vi "characterisation.vi"   [LabVIEW 2019]
uses:
  Shared VIs/ModelSpecific/ETHMikeModel.ctl
  Shared VIs/ModelSpecific/ReadOnlyGlobalActions.ctl
types:
  T1 = typedef "ReadOnlyGlobalActions.ctl" = enum16{"Initialize", "Read", "Write"}
  T2 = typedef "ETHMikeModel.ctl" = enum16{"ETH Mike #1", "ETH Mike #2", "ETH Mike #3", "ETH Mike #4", "ETH MIKE #5"}
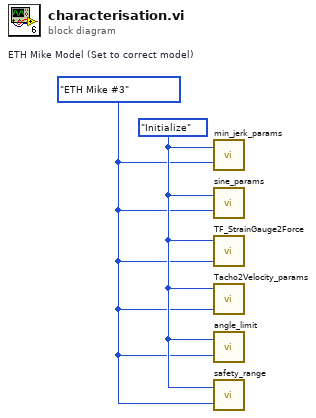
[diagram p0: block diagram]
diagram:
  w2 = ReadOnlyGlobalActions."Initialize" ("Action (Read)")
  w1 = ETHMikeModel."ETH Mike #3"  # ETH Mike Model (Set to correct model)
  n1 = call "min_jerk_params.vi"("Action (Read)"=w2, "ETH Mike Model"=w1) -> ()  [unwired: 17 in, 1 out]
  n2 = call "sine_params.vi"("Action (Read)"=w2, "ETH Mike Model"=w1) -> ()  [unwired: 17 in, 1 out]
  n3 = call "TF_StrainGauge2Force.vi"("Action (Read)"=w2, "ETH Mike Model"=w1) -> ()  [unwired: 3 in, 1 out]
  n4 = call "Tacho2Velocity_params.vi"("Action (Read)"=w2, "ETH Mike Model"=w1) -> ()  [unwired: 3 in, 1 out]
  n5 = call "angle_limit.vi"("ETH Mike Model"=w1, "Action (Read)"=w2) -> ()  [unwired: 1 out]
  n6 = call "safety_range.vi"("ETH Mike Model"=w1, "Action (Read)"=w2) -> ()  [unwired: 1 out]
